vi "Data Logger.vi"() -> ()   [LabVIEW 2020]
panel:
  in  "Table Control":string[][](table)
  out "Temperature Chart":dbl(graph)
  out "Humidity Chart":dbl(graph)
  out "Humidity / %":dbl(knob) scale=0.0..100.0
  in  "VISA resource name":refnum<visa-resource-name>
  out "Temperature / °C":dbl(slide) scale=0.0..100.0
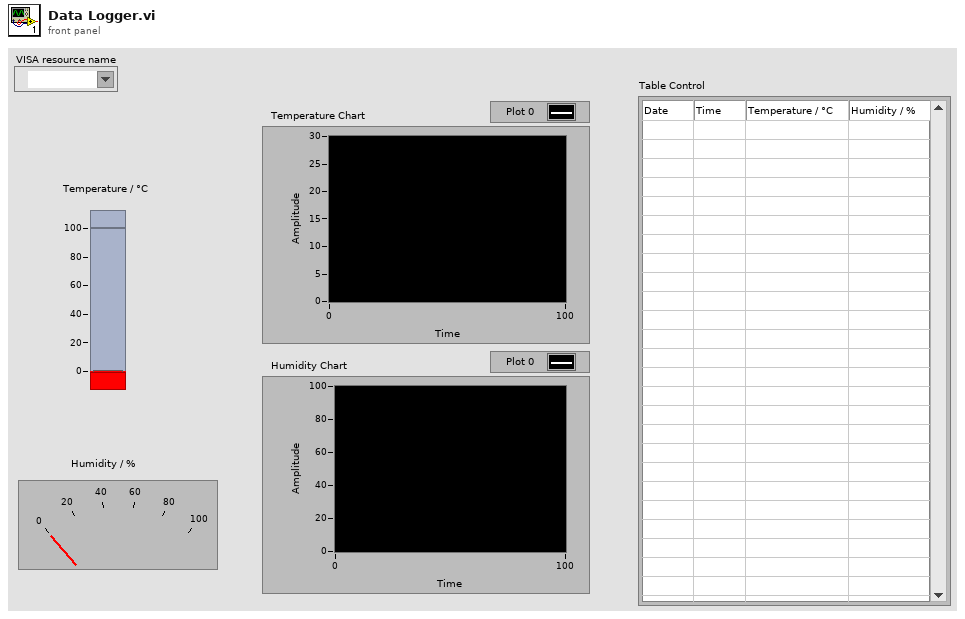
[diagram p1: front panel]
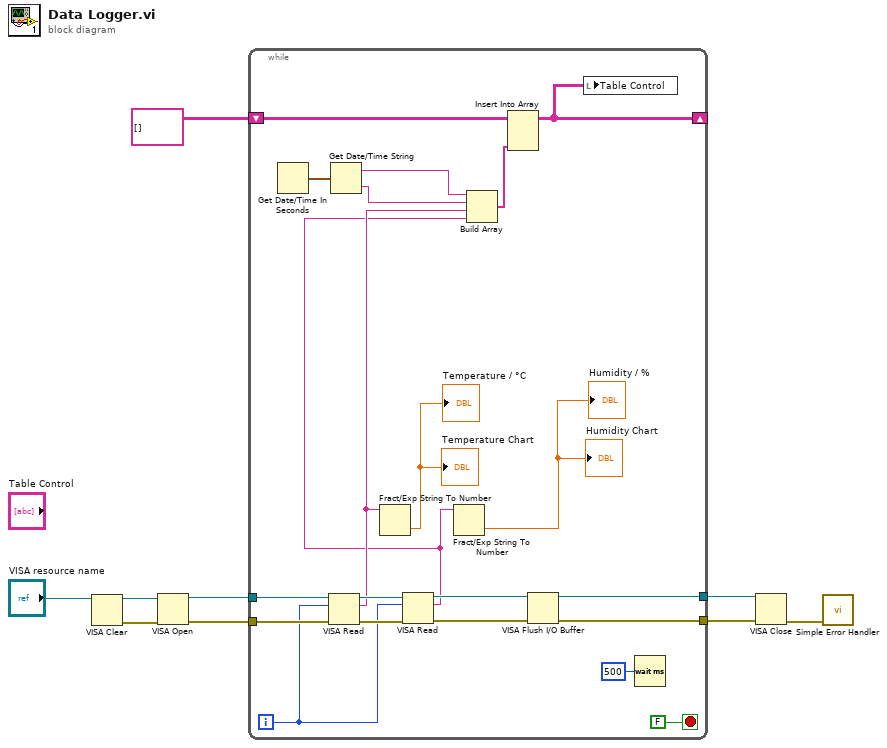
[diagram p0: block diagram]
diagram:
  n1 = VISA Clear(VISA resource name="VISA resource name") -> (VISA resource name out=w7:refnum<visa-resource-name>, error out=w6:errorcluster)  [unwired: 1 in]
  n2 = VISA Open(error in (no error)=w6, VISA resource name=w7) -> (VISA resource name=w9:refnum<visa-resource-name>, error out=w8:errorcluster)  [unwired: 3 in]
  n3 = while {
    tunnel: w9 -> [w26]
    tunnel: w8 -> [w25]
    tunnel: [w24] -> w5
    tunnel: [w23] -> w4
    shift-right: [w18] -> _
    shift-left: string[][] [] -> [w19]
    i -> [w22]
    stop <- FALSE stop-if-true
    n4 = Get Date/Time In Seconds() -> (seconds since 1Jan1904=w17:timestamp)
    n5 = VISA Read(VISA resource name=w26, byte count=w22, error in (no error)=w25) -> (VISA resource name out=w30:refnum<visa-resource-name>, read buffer=w14:string, error out=w29:errorcluster)  [unwired: 1 out]
    n6 = Get Date/Time String(seconds (now)=w17) -> (date string=w16:string, time string=w15:string)  [unwired: 2 in]
    n7 = Fract/Exp String To Number(string=w14) -> (number=→"Temperature / °C" →"Temperature Chart":dbl)  [unwired: 3 in, 1 out]
    n8 = VISA Read(VISA resource name=w30, byte count=w22, error in (no error)=w29) -> (VISA resource name out=w28:refnum<visa-resource-name>, read buffer=w13:string, error out=w27:errorcluster)  [unwired: 1 out]
    n9 = Fract/Exp String To Number(string=w13) -> (number=→"Humidity / %" →"Humidity Chart":dbl)  [unwired: 3 in, 1 out]
    n10 = Build Array(w16, w15, w14, w13) -> (w12:string[])
    n11 = Insert Into Array(array=w19, new element=w12) -> (w18:string[][])  [unwired: 2 in]
    n12 = VISA Flush I/O Buffer(VISA resource name=w28, error in (no error)=w27) -> (VISA resource name out=w24:refnum<visa-resource-name>, error out=w23:errorcluster)  [unwired: 1 in]
    n13 = local write "Table Control"(w18) -> ()
    n14 = Wait (ms)(milliseconds to wait=u32 500) -> ()  [unwired: 1 out]
  }
  n15 = VISA Close(VISA resource name=w5, error in (no error)=w4) -> (error out=w3:errorcluster)
  n16 = call <vilib>:"Simple Error Handler.vi"("error in (no error)"=w3) -> ()  [unwired: 4 in, 5 out]
